vi "NormaliseProfile.vi"(5 "ResampleHeights":dbl[](array[numeric])=[25.4, 38.1, 50.8, 76.2, 101.6, 127.0, 152.4, 203.2, 254.0, 304.8, 406.4, 508.0, 609.6, 812.8, 1219.2, 1524.0], 6 "Zref":dbl=508.0 min=0.0, 7 "ResampleToN":i32, 8 "Normalise?":bool=TRUE, 10 "UzClusterIn":cluster{dbl[], dbl[]}, 11 "Resampler":T1) -> (1 "U(Zref)":dbl, 3 "UzClusterOutput":cluster{dbl[], dbl[]})   [LabVIEW 2021]
uses:
  Resampler.ctl
  <vilib>/Analysis/NI_AALPro.lvlib
  <vilib>/gmath/NI_Gmath.lvlib
panel:
  in  "Interpolation":i32(ring)=1 items=["nearest", "linear", "spline", "cubic Hermite", "Lagrange"]
  out "UzClusterNormalisedResampled":cluster{dbl[], dbl[]}
  out "UzClusterNormalised":cluster{dbl[], dbl[]}
  in  "binTolerance":dbl=10.0
  out "firstBelow":dbl
  out "firstAbove":dbl
  out "XY Graph":cluster{dbl[], dbl[]}[](graph)
  # "Fit using values at  measurement Z heights"
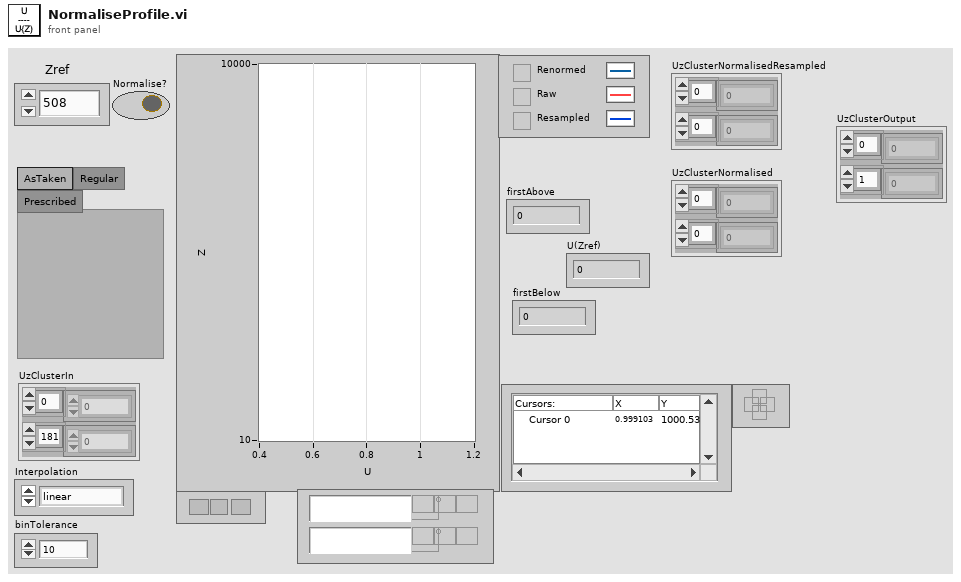
[diagram p1: front panel]
types:
  T1 = typedef "Resampler.ctl" = enum32{"AsTaken", "Regular", "Prescribed"}
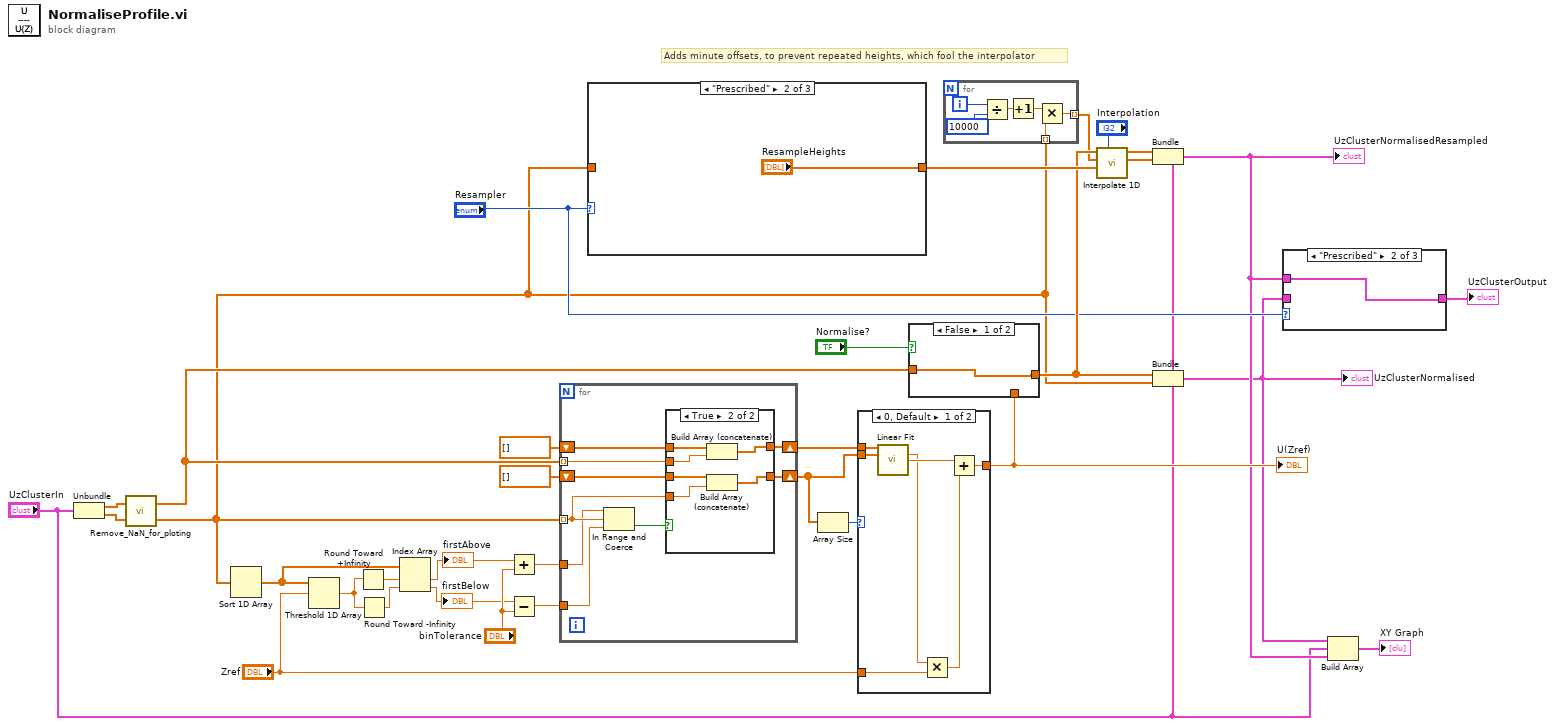
[diagram p0: block diagram]
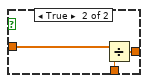
[diagram p2: hidden frame]
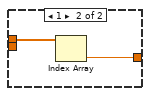
[diagram p5: hidden frame]
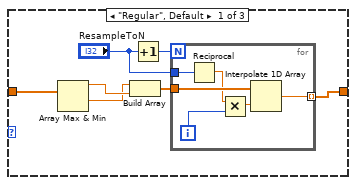
[diagram p6: hidden frame]
diagram:
  # "Adds minute offsets, to prevent repeated heights, which fool the interpolator"
  n1 = Unbundle("UzClusterIn") -> (w20:dbl[], w21:dbl[])
  n2 = call "Remove_NaN_for_ploting.vi"("Array 2"=w21, "Array 1"=w20) -> ("Array 2 Out"=w7:dbl[], "Array 1 Out"=w19:dbl[])
  n3 = Sort 1D Array(array=w7) -> (sorted array=w32:dbl[])
  n4 = Threshold 1D Array(2:"Zref", 3:w32) -> (0:w33:dbl)  [unwired: 1 in]
  n5 = Round Toward +Infinity(x=w33) -> (ceil(x): smallest int >= x=w31:dbl)
  n6 = Round Toward -Infinity(1:w33) -> (0:w30:dbl)
  n7 = Index Array(array=w32, index #1=w31, index #2=w30) -> (element #1=w14:dbl, element #2=w13:dbl)
  "firstAbove" <- w14
  "firstBelow" <- w13
  n8 = Add(x=w14, y="binTolerance") -> (x+y=w28:dbl)
  n9 = Subtract(x=w13, y="binTolerance") -> (x-y=w27:dbl)
  n10 = for {
    tunnel: w19 -> [w41] mode=indexing
    tunnel: w7 -> [w42] mode=indexing
    tunnel: w28 -> [w36]
    tunnel: w27 -> [w35]
    shift-right: [w40] -> w26
    shift-left: dbl[] [] -> [w39]
    shift-right: [w37] -> w9
    shift-left: dbl[] [] -> [w38]
    n11 = In Range and Coerce(upper limit=w36, x=w42, lower limit=w35) -> (In Range?=w34:bool)  [unwired: 1 out]
    n12 = case shown="True" w34 {
      tunnel: w42 -> [_ w50]
      tunnel: w41 -> [_ w49]
      tunnel: [w44 w48] -> w40
      tunnel: w39 -> [w44 w47]
      tunnel: w38 -> [w43 w46]
      tunnel: [w43 w45] -> w37
      frame False {
      }
      frame True {
        n13 = Build Array (concatenate)(w47, w49) -> (w48:dbl[])
        n14 = Build Array (concatenate)(w46, w50) -> (w45:dbl[])
      }
    }
  }
  n15 = case shown="\"Prescribed\"" "Resampler" {
    tunnel: [w53 "ResampleHeights" w65] -> w16
    tunnel: w7 -> [w51 _ w65]
    frame "Regular", Default {
      n16 = Array Max & Min(array=w51) -> (max value=w55:dbl, min value=w54:dbl)  [unwired: 2 out]
      n17 = Build Array(w54, w55) -> (w57:dbl[])
      n18 = Increment(x="ResampleToN") -> (x+1=w52:i32)
      n19 = for {
        N: w52 -> [_]
        tunnel: w57 -> [w63]
        tunnel: "ResampleToN" -> [w62]
        tunnel: [w59] -> w53 mode=indexing
        i -> [w58]
        n20 = Reciprocal(x=w62) -> (1/x=w60:dbl)
        n21 = Multiply(x=w60, y=w58) -> (x*y=w61:dbl)
        n22 = Interpolate 1D Array(1:w61, 2:w63) -> (0:w59:dbl)
      }
    }
    frame "Prescribed" {
    }
    frame "AsTaken" {
    }
  }
  n23 = Array Size(array=w9) -> (size(s)=w12:i32)
  n24 = case shown="0, Default" w12 {
    tunnel: w26 -> [w72 w74]
    tunnel: "Zref" -> [w69 _]
    tunnel: [w67 w73] -> w25
    tunnel: w9 -> [w66 _]
    frame 0, Default {
      n25 = call <vilib>:"Linear Fit.vi"("Y"=w72, "X"=w66) -> ("slope"=w70:dbl, "intercept"=w71:dbl)  [unwired: 9 in, 3 out]
      n26 = Multiply(x=w70, y=w69) -> (x*y=w68:dbl)
      n27 = Add(x=w71, y=w68) -> (x+y=w67:dbl)
    }
    frame 1 {
      n28 = Index Array(array=w74) -> (element=w73:dbl)  [unwired: 1 in]
    }
  }
  "U(Zref)" <- w25
  n29 = case shown="False" "Normalise?" {
    tunnel: w25 -> [_ w78]
    tunnel: w19 -> [w75 w77]
    tunnel: [w75 w76] -> w15
    frame False {
    }
    frame True {
      n30 = Divide(x=w77, y=w78) -> (x/y=w76:dbl[])
    }
  }
  n31 = for {
    tunnel: [w79] -> w8 mode=indexing
    tunnel: w7 -> [w80] mode=indexing
    i -> [w84]
    n32 = Divide(x=w84, y=10000) -> (x/y=w82:dbl)
    n33 = Increment(x=w82) -> (x+1=w81:dbl)
    n34 = Multiply(x=w81, y=w80) -> (x*y=w79:dbl)
  }
  n35 = call <vilib>:"Interpolate 1D.vi"("method"="Interpolation", "xi"=w16, "X"=w8, "Y"=w15) -> ("xi used"=w6:dbl[], "yi"=w17:dbl[])  [unwired: 5 in, 1 out]
  n36 = Bundle(cluster="UzClusterIn", w17, w6) -> (w4:cluster{dbl[], dbl[]})
  "UzClusterNormalisedResampled" <- w4
  n37 = Bundle(cluster="UzClusterIn", w15, w7) -> (w2:cluster{dbl[], dbl[]})
  "UzClusterNormalised" <- w2
  n38 = case shown="\"Prescribed\"" "Resampler" {
    tunnel: [w85 w86 w87] -> w10
    tunnel: w4 -> [w85 w86 _]
    tunnel: w2 -> [_ _ w87]
    frame "Regular", Default {
    }
    frame "Prescribed" {
    }
    frame "AsTaken" {
    }
  }
  "UzClusterOutput" <- w10
  n39 = Build Array(w2, "UzClusterIn", w4) -> (→"XY Graph":cluster{dbl[], dbl[]}[])
